vi "Target Write Lever Arm Polynomial to Disk.vi"() -> ()   [LabVIEW 2018, in "COBRA Prosthesis Model Library.lvlib"]
uses:
  <vilib>/Analysis/polynomials.llb/1D Polynomial Evaluation (DBL).vi
  COBRA Prosthesis Model Library.lvlib
  <vilib>/Analysis/NI_AALPro.lvlib
panel:
  in  "Lever Arm Polynomial Coefficients":dbl[](array[numeric])
  in  "Stop":bool
  in  "Save Coefficients":bool
  in  "Update Coefficients":bool
  out "Lever Arm Plot":cluster{"X":dbl, "Y":dbl}[](graph)
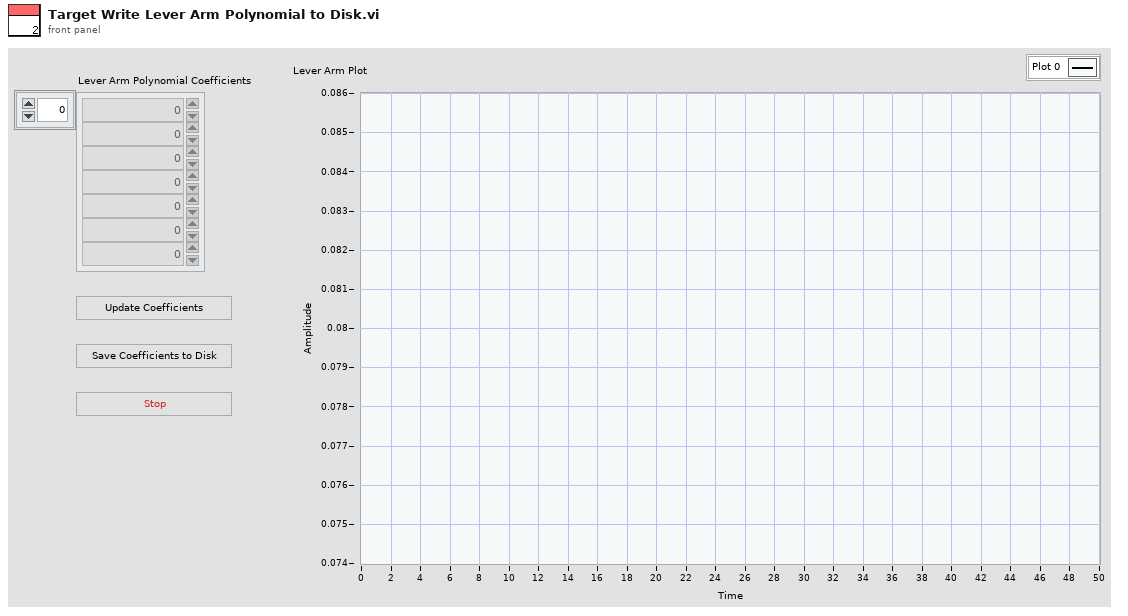
[diagram p1: front panel]
types:
  T1 = enum16{"open", "open or create", "create or replace", "create", "open (read-only)"}
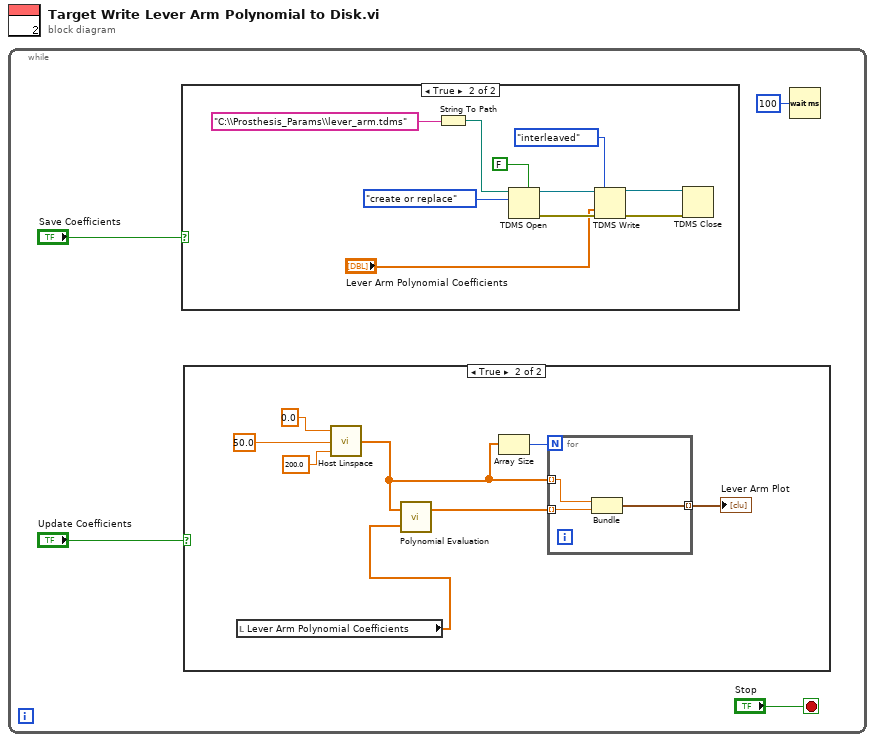
[diagram p0: block diagram]
diagram:
  n1 = while {
    stop <- "Stop" stop-if-true
    n2 = case shown="True" "Save Coefficients" {
      frame False {
      }
      frame True {
        n3 = String To Path(string="C:\\Prosthesis_Params\\lever_arm.tdms") -> (path=w22:path)
        n4 = TDMS Open(5:FALSE ("create index file? (T)"), 10:T1."create or replace" ("operation (0:open)"), 11:w22) -> (0:w18:errorcluster, 3:w21:refnum<k34>)  [unwired: 4 in]
        n5 = TDMS Write(0:w21, 1:enum16{"decimated", "interleaved"}."interleaved" ("data layout (0:decimated)"), 9:"Lever Arm Polynomial Coefficients", 11:w18) -> (4:w19:refnum<k34>, 15:w20:errorcluster)  [unwired: 2 in, 2 out]
        n6 = TDMS Close(8:w20, 11:w19) -> ()  [unwired: 2 out]
      }
    }
    n7 = case shown="True" "Update Coefficients" {
      frame False {
      }
      frame True {
        n8 = local read "Lever Arm Polynomial Coefficients"() -> (w5:dbl[])
        n9 = call "Host Linspace.vi"("NumElements"=200.0, "End"=50.0, "Start"=0.0) -> ("Array"=w9:dbl[])
        n10 = call-poly <vilib>:"Polynomial Evaluation.vi"("P(x)"=w5, "A"=w9) -> ("P(A)"=w11:dbl[])  [unwired: 1 out]
        n11 = Array Size(array=w9) -> (size(s)=w12:i32)
        n12 = for {
          N: w12 -> [_]
          tunnel: w11 -> [w14] mode=indexing
          tunnel: w9 -> [w15] mode=indexing
          tunnel: [w13] -> w10 mode=indexing
          n13 = Bundle("Numeric"=w15, "p(x)"=w14) -> (w13:cluster{"Numeric":dbl, "p(x)":dbl})  [unwired: 1 in]
        }
        "Lever Arm Plot" <- w10
      }
    }
    n14 = Wait (ms)(milliseconds to wait=u32 100) -> ()  [unwired: 1 out]
  }
